vi "RobotDriveOpen6MotorWithTalonSR.vi"(0 "Left Motor 1":T1, 1 "Left Motor 2":T1, 2 "Left Motor 3":T1, 3 "Right Motor 1":T1, 4 "Right Motor 2":T1, 5 "Right Motor 3":T1, 7 "error in (no error)":errorcluster, 8 "Left Motor 1 Inverted":bool, 9 "Right Motor 1 Inverted":bool, 10 "Left Motor 2 Inverted":bool, 11 "Right Motor 2 Inverted":bool, 12 "Left Motor 3 Inverted":bool, 13 "Right Motor 3 Inverted":bool) -> (20 "RobotDriveDevRef":T2={"DevStatus"={"status"=FALSE, "code"=0, "source"=""}, "Motors[]"=[], "Square Inputs"=FALSE, "Max Output"=1.0}, 27 "error out":errorcluster)   [LabVIEW 2016]
doc: "Opens a reference to the robot drive for a four-motor robot using VictorSP motor controllers.\n\nThis software is licensed. Open the labview\\readme\\WPI Robotics Library Open Source License.txt file for more information."
uses:
  <vilib>/Rock Robotics/WPI/RobotDrive/WPI_RobotDriveDevRef.ctl
  <vilib>/Rock Robotics/WPI/MotorControl/WPI_MotorControlDeviceRef.ctl
  <vilib>/Rock Robotics/WPI/MotorControl/WPI_MotorControlType.ctl
  <vilib>/Rock Robotics/SystemInterfaces/DIO/FPGA_DIOPWMChannel.ctl
  <vilib>/Rock Robotics/WPI/PWM/WPI_PWMDeadband.ctl
  <vilib>/Rock Robotics/WPI/SafetyOutput/WPI_SafetyOutputConfigMenu.ctl
  <vilib>/Rock Robotics/WPI/MotorControl/WPI_MotorControlOpen Talon.vi
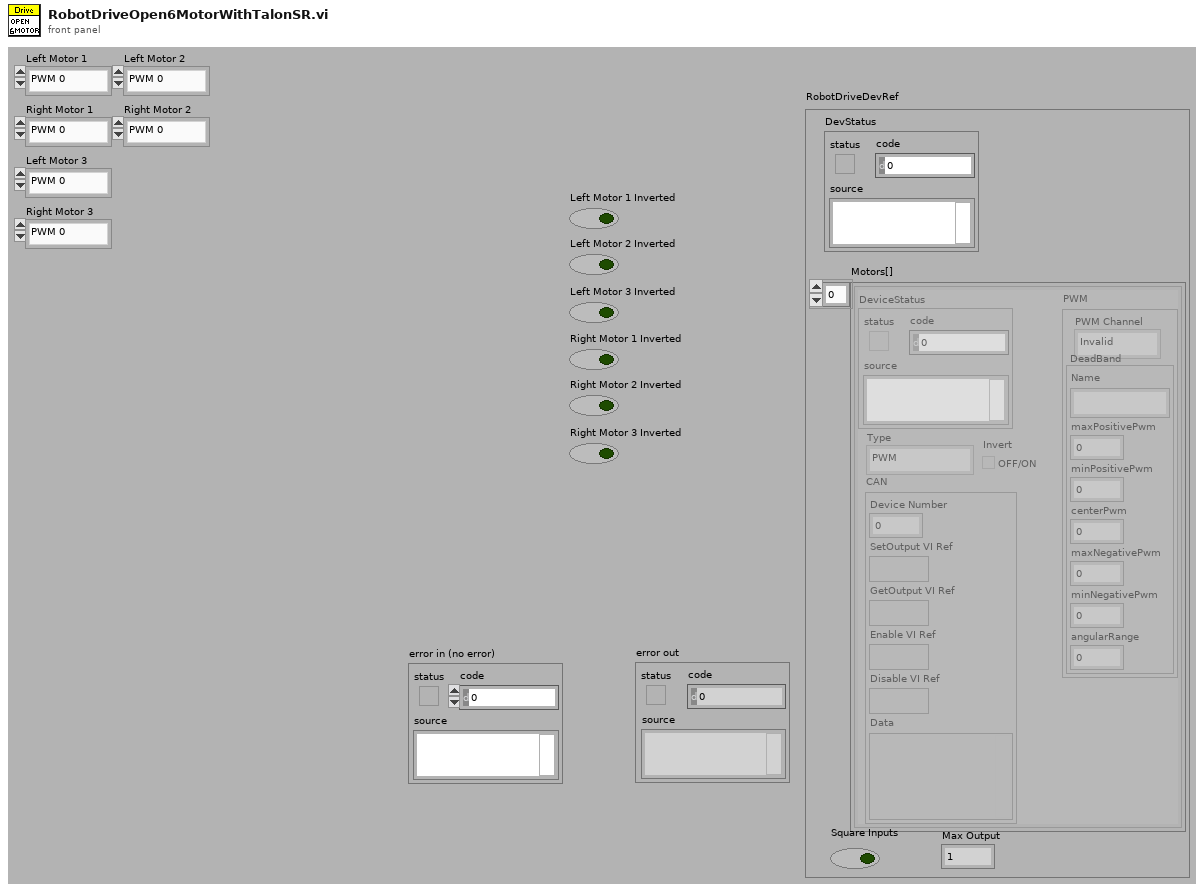
[diagram p1: front panel]
types:
  T1 = typedef "FPGA_DIOPWMChannel.ctl" = enum8{"PWM 0", "PWM 1", "PWM 2", "PWM 3", "PWM 4", "PWM 5", "PWM 6", "PWM 7", "PWM 8", "PWM 9", "PWM MXP 0", "PWM MXP 1", "PWM MXP 2", "PWM MXP 3", "PWM MXP 4", "PWM MXP 5", "PWM MXP 6", "PWM MXP 7", "PWM MXP 8", "PWM MXP 9", "Invalid"}
  T2 = typedef "WPI_RobotDriveDevRef.ctl" = cluster{"DevStatus":errorcluster, "Motors[]":T3[], "Square Inputs":bool, "Max Output":dbl}
  T3 = typedef "WPI_MotorControlDeviceRef.ctl" = cluster{"DeviceStatus":errorcluster, "Type":T4, "PWM":cluster{"PWM Channel":T1, "DeadBand":T5}, "CAN":cluster{"Device Number":u8, "SetOutput VI Ref":variant, "GetOutput VI Ref":variant, "Enable VI Ref":variant, "Disable VI Ref":variant, "Data":variant}, "Invert":bool}
  T4 = typedef "WPI_MotorControlType.ctl" = enum16{"PWM", "CAN"}
  T5 = typedef "WPI_PWMDeadband.ctl" = cluster{"Name":string, "maxPositivePwm":i32, "minPositivePwm":i32, "centerPwm":i32, "maxNegativePwm":i32, "minNegativePwm":i32, "angularRange":u16}
  T6 = typedef "WPI_SafetyOutputConfigMenu.ctl" = enum16{"Enable", "Disable"}
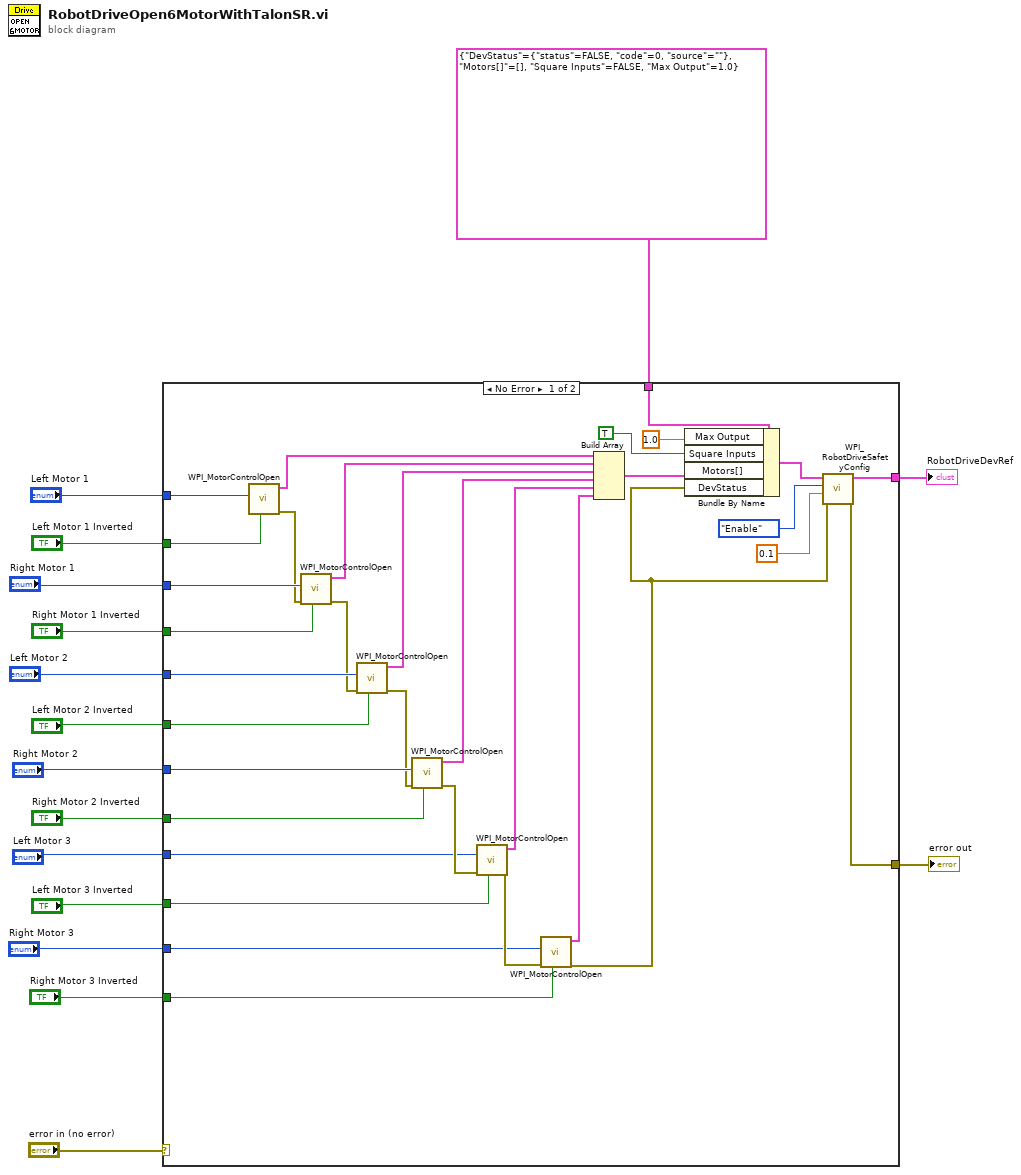
[diagram p0: block diagram]
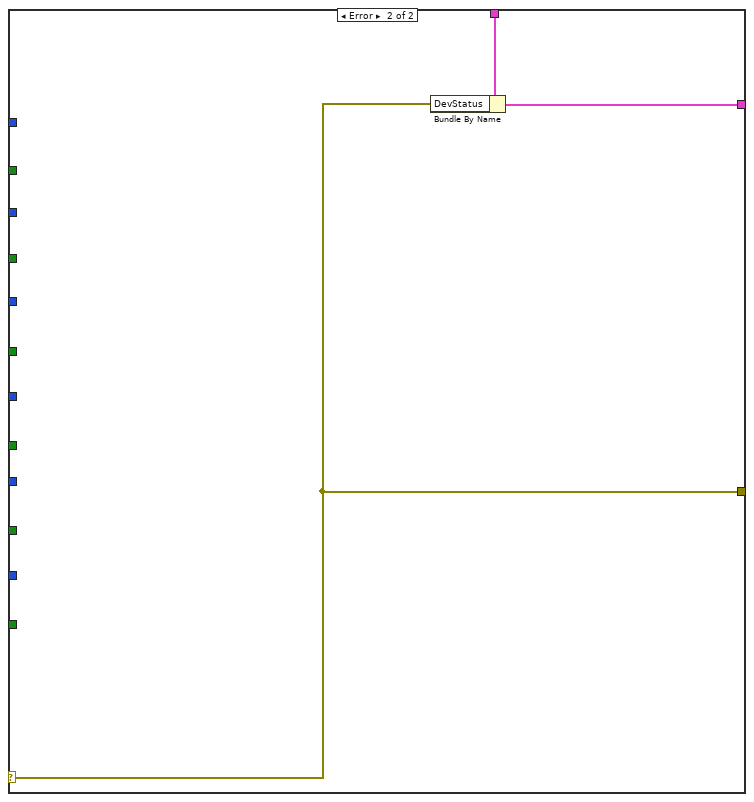
[diagram p2: hidden frame]
diagram:
  n1 = case shown="No Error" "error in (no error)" {
    selector: "error in (no error)" -> [_ w50]
    tunnel: [w29 w51] -> w16
    tunnel: T2 {"DevStatus"={"status"=FALSE, "code"=0, "source"=""}, "Motors[]"=[], "Square Inputs"=FALSE, "Max Output"=1.0} ("RobotDriveDevRef") -> [w49 w52]
    tunnel: "Right Motor 2" -> [w45 _]
    tunnel: "Left Motor 2" -> [w46 _]
    tunnel: "Right Motor 1" -> [w47 _]
    tunnel: "Left Motor 1 Inverted" -> [w36 _]
    tunnel: "Right Motor 1 Inverted" -> [w35 _]
    tunnel: "Right Motor 2 Inverted" -> [w33 _]
    tunnel: "Left Motor 2 Inverted" -> [w34 _]
    tunnel: [w30 w50] -> w9
    tunnel: "Left Motor 3" -> [w22 _]
    tunnel: "Left Motor 3 Inverted" -> [w20 _]
    tunnel: "Right Motor 3" -> [w21 _]
    tunnel: "Right Motor 3 Inverted" -> [w19 _]
    tunnel: "Left Motor 1" -> [w17 _]
    frame No Error {
      n2 = call-poly <vilib>:"WPI_MotorControlOpen.vi"("Invert"=w36, "PWM Channel"=w17) -> ("error out"=w38:errorcluster, "MotorControlDeviceRef"=w44:T3)  [unwired: 2 in, 6 out]
      n3 = call-poly <vilib>:"WPI_MotorControlOpen.vi"("Invert"=w35, "error in (no error)"=w38, "PWM Channel"=w47) -> ("error out"=w39:errorcluster, "MotorControlDeviceRef"=w43:T3)  [unwired: 1 in, 6 out]
      n4 = call-poly <vilib>:"WPI_MotorControlOpen.vi"("Invert"=w34, "error in (no error)"=w39, "PWM Channel"=w46) -> ("error out"=w40:errorcluster, "MotorControlDeviceRef"=w42:T3)  [unwired: 1 in, 6 out]
      n5 = call-poly <vilib>:"WPI_MotorControlOpen.vi"("Invert"=w33, "error in (no error)"=w40, "PWM Channel"=w45) -> ("error out"=w26:errorcluster, "MotorControlDeviceRef"=w41:T3)  [unwired: 1 in, 6 out]
      n6 = call-poly <vilib>:"WPI_MotorControlOpen.vi"("Invert"=w20, "error in (no error)"=w26, "PWM Channel"=w22) -> ("error out"=w25:errorcluster, "MotorControlDeviceRef"=w24:T3)  [unwired: 1 in, 6 out]
      n7 = call-poly <vilib>:"WPI_MotorControlOpen.vi"("Invert"=w19, "error in (no error)"=w25, "PWM Channel"=w21) -> ("error out"=w18:errorcluster, "MotorControlDeviceRef"=w23:T3)  [unwired: 1 in, 6 out]
      n8 = Build Array(w44, w43, w42, w41, w24, w23) -> (w37:T3[])
      n9 = Bundle By Name(cluster=w49, "Max Output"=1.0, "Square Inputs"=TRUE ("DestroyPWM?"), "Motors[]"=w37, "DevStatus"=w18) -> (w31:T2)
      n10 = call <vilib>:"WPI_RobotDriveSafetyConfig.vi"("error in (no error)"=w18, "timeout (s)"=0.1, "mode"=WPI_SafetyOutputConfigMenu."Enable", "RobotDriveDevRef"=w31) -> ("error out"=w30:errorcluster, "RobotDriveDevRef"=w29:T2)  [unwired: 6 out]
    }
    frame Error {
      n11 = Bundle By Name(cluster=w52, "DevStatus"=w50) -> (w51:T2)
    }
  }
  "RobotDriveDevRef" <- w16
  "error out" <- w9
